vi "Get_file_1st_element.vi"(11 "File Path":path) -> (3 "First element":dbl format="%.2f")   [LabVIEW 2020]
panel:
  out "element":string
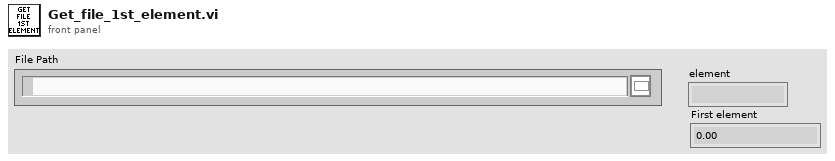
[diagram p1: front panel]
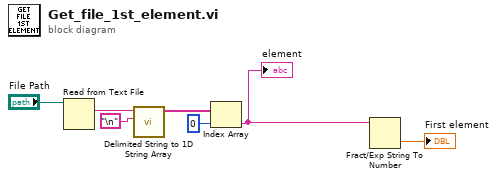
[diagram p0: block diagram]
diagram:
  n1 = Read from Text File(file (use dialog)="File Path") -> (text=w6:string)  [unwired: 3 in, 3 out]
  n2 = call <vilib>:"Delimited String to 1D String Array.vi"("delimiter"="\n", "delimited string"=w6) -> ("string array"=w4:string[])  [unwired: 9 in]
  n3 = Index Array(array=w4, index=0) -> (element=w2:string)
  "element" <- w2
  n4 = Fract/Exp String To Number(string=w2) -> (number=→"First element":dbl)  [unwired: 3 in, 1 out]
